vi "NI VeriStand - Lock Workspace File.vi"(8 "error in (no error)":errorcluster, 9 "New Password":string, 10 "Old Password (\"\")":string, 11 "WorkspaceManager in":T1) -> (0 "error out":errorcluster, 3 "WorkspaceManager out":T1)   [LabVIEW 2020, in "NI_VS Workspace ExecutionAPI.lvlib"]
doc: "Locks a currently running workspace file with a password to prevent unauthorized shutdown of the workspace file."
uses:
  <vilib>/NI VeriStand/Execution/Workspace/NI_VS Workspace ExecutionAPI.lvlib
  <vilib>/NI VeriStand/Execution/Workspace/WorkspaceAPI.ctl
  NationalInstruments.VeriStand.ClientAPI
panel:
  # "This VI has been deprecated in favor of NI VeriStand - Lock Connection.vi."
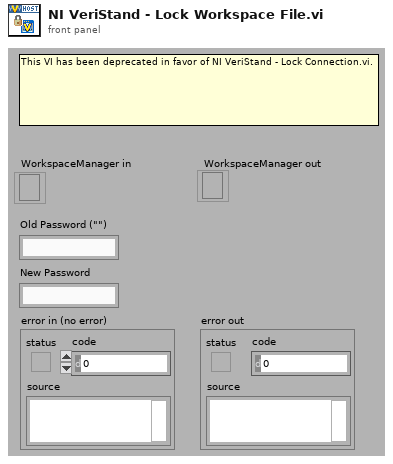
[diagram p1: front panel]
types:
  T1 = typedef "NI_VS Workspace ExecutionAPI.lvlib/WorkspaceAPI.ctl" = refnum<k24>
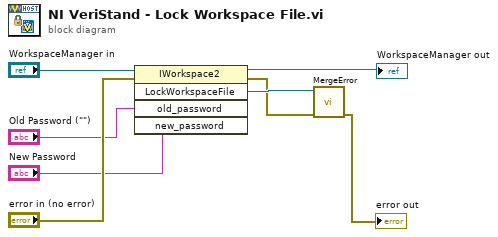
[diagram p0: block diagram]
diagram:
  n1 = invoke class="IWorkspace2" method="LockWorkspaceFile"(reference="WorkspaceManager in", error in="error in (no error)", "old_password"="Old Password (\"\")", "new_password"="New Password") -> (reference out=→"WorkspaceManager out":T1, error out=w3:errorcluster, "LockWorkspaceFile"=w4:refnum<k24>)  [unwired: 1 in, 2 out]
  n2 = call <vilib>:"MergeError.vi"("error in (no error)"=w3, "Error"=w4) -> ("error out"=→"error out":errorcluster)  [unwired: 9 out]
